vi "Imaging.vi"() -> ()   [LabVIEW 2015]
uses:
  <userlib>/atmcd64d.llb/Error Code Enum typedef.ctl
  <userlib>/atmcd64d.llb/AcquisitionMode_mode typedef.ctl
  <userlib>/atmcd64d.llb/HSSpeed_type typedef.ctl
  <userlib>/atmcd64d.llb/ReadMode_mode typedef.ctl
  <userlib>/atmcd64d.llb/TriggerMode_mode typedef.ctl
  <userlib>/atmcd64d.llb/Shutter_type typedef.ctl
  <userlib>/atmcd64d.llb/Shutter_mode typedef.ctl
  LiveImage.vi
panel:
  out "Intensity Graph":i32[][](graph)
  in  "Live Acquisition Start":bool
  in  "Set HS Speed":u16(ring) items=["17", "10", "5", "1"]
  out "#VS Speeds":i32
  in  "Acquisition Mode":T1=enum."Single Scan"
  in  "stop":bool
  out "status":T2
  out "minTemp":i32
  out "maxTemp":i32
  out "ypixels":i32
  out "xpixels":i32
  out "temperature":sgl
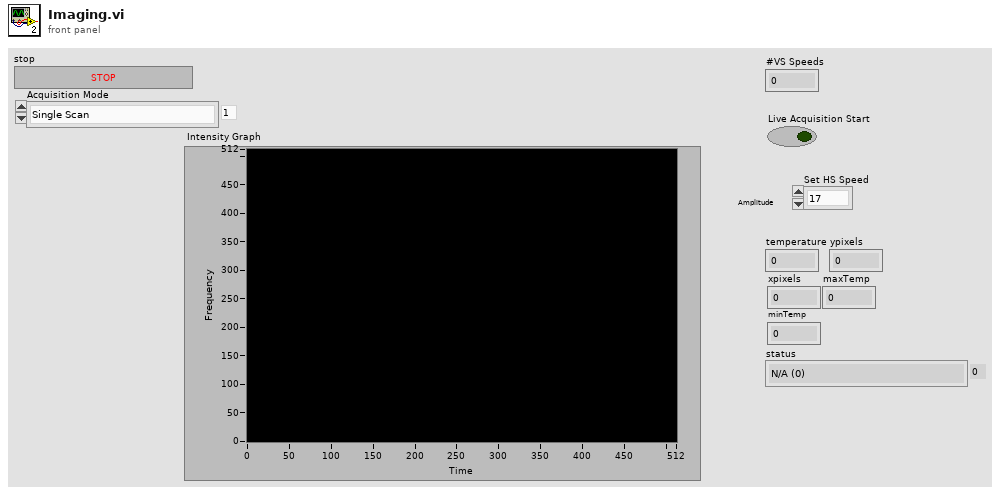
[diagram p1: front panel]
types:
  T1 = typedef "AcquisitionMode_mode typedef.ctl" = enum16{"Reserved (0)", "Single Scan", "Accumulate", "Kinetics", "Fast Kinetics", "Run Till Abort", "Reserved (6)", "Reserved (7)", "Reserved (8)", "Time Delayed Integration"}
  T2 = typedef "Error Code Enum typedef.ctl" = enum32{"N/A (0)", "DRV_ERROR_CODES", "DRV_SUCCESS", "DRV_VXDNOTINSTALLED", "DRV_ERROR_SCAN", "DRV_ERROR_CHECK_SUM", "DRV_ERROR_FILELOAD", "DRV_UNKNOWN_FUNC", "DRV_ERROR_VXD_INIT", "DRV_ERROR_ADDRESS", "DRV_ERROR_PAGELOCK", "DRV_ERROR_PAGEUNLOCK", "DRV_ERROR_BOARDTEST", "DRV_ERROR_ACK", "DRV_ERROR_UP_FIFO", "DRV_ERROR_PATTERN", "N/A (16)", "DRV_ACQUISITION_ERRORS", "DRV_ACQ_BUFFER", "DRV_ACQ_DOWNFIFO_FULL", "DRV_PROC_UNKONWN_INSTRUCTION", "DRV_ILLEGAL_OP_CODE", "DRV_KINETIC_TIME_NOT_MET", "DRV_ACCUM_TIME_NOT_MET", "DRV_NO_NEW_DATA", "N/A (25)", "DRV_SPOOLERROR", "N/A (27)", "N/A (28)", "N/A (29)", "N/A (30)", "N/A (31)", "N/A (32)", "DRV_TEMPERATURE_CODES", "DRV_TEMPERATURE_OFF", "DRV_TEMPERATURE_NOT_STABILIZED", "DRV_TEMPERATURE_STABILIZED", "DRV_TEMPERATURE_NOT_REACHED", "DRV_TEMPERATURE_OUT_RANGE", "DRV_TEMPERATURE_NOT_SUPPORTED", "DRV_TEMPERATURE_DRIFT", "N/A (41)", "N/A (42)", "N/A (43)", "N/A (44)", "N/A (45)", "N/A (46)", "N/A (47)", "N/A (48)", "DRV_GENERAL_ERRORS", "DRV_INVALID_AUX", "DRV_COF_NOTLOADED", "DRV_FPGAPROG", "DRV_FLEXERROR", "DRV_GPIBERROR", "N/A (55)", "N/A (56)", "N/A (57)", "N/A (58)", "N/A (59)", "N/A (60)", "N/A (61)", "N/A (62)", "N/A (63)", "DRV_DATATYPE", "DRV_DRIVER_ERRORS", "DRV_P1INVALID", "DRV_P2INVALID", "DRV_P3INVALID", "DRV_P4INVALID", "DRV_INIERROR", "DRV_COFERROR", "DRV_ACQUIRING", "DRV_IDLE", "DRV_TEMPCYCLE", "DRV_NOT_INITIALIZED", "DRV_P5INVALID", "DRV_P6INVALID", "DRV_INVALID_MODE", "DRV_INVALID_FILTER", "DRV_I2CERRORS", "DRV_I2CDEVNOTFOUND", "DRV_I2CTIMEOUT", "DRV_P7INVALID", "N/A (84)", "N/A (85)", "N/A (86)", "N/A (87)", "N/A (88)", "N/A (89)", "DRV_IOCERROR", "DRV_VRMVERSIONERROR"}
  T3 = typedef "Shutter_mode typedef.ctl" = enum16{"Auto", "Open", "Close", "N/A (3)", "Open FVB Series", "Open Any Series"}
  T4 = typedef "Shutter_type typedef.ctl" = enum16{"TTL Low", "TTL High"}
  T5 = typedef "TriggerMode_mode typedef.ctl" = enum16{"Internal", "External", "N/A (2)", "N/A (3)", "N/A (4)", "N/A (5)", "External Start", "External Exposure (Bulb)", "N/A (8)", "External FVB EM", "Software", "N/A (11)", "External Charge Shifting"}
  T6 = typedef "ReadMode_mode typedef.ctl" = enum16{"Full Vertical Binning", "Multi-Track", "Random-Track", "Single-Track", "Image"}
  T7 = typedef "HSSpeed_type typedef.ctl" = enum16{"EM Amp", "Conventional Amp"}
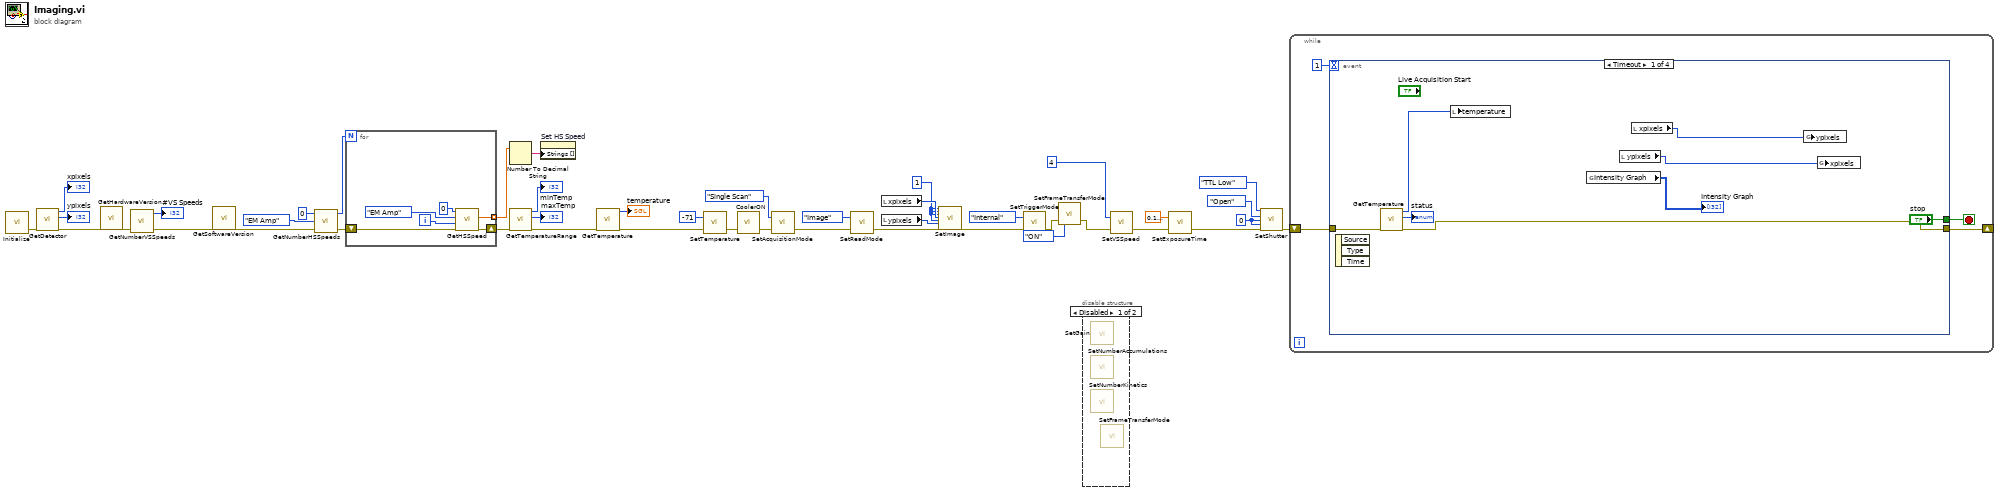
[diagram p0: block diagram]
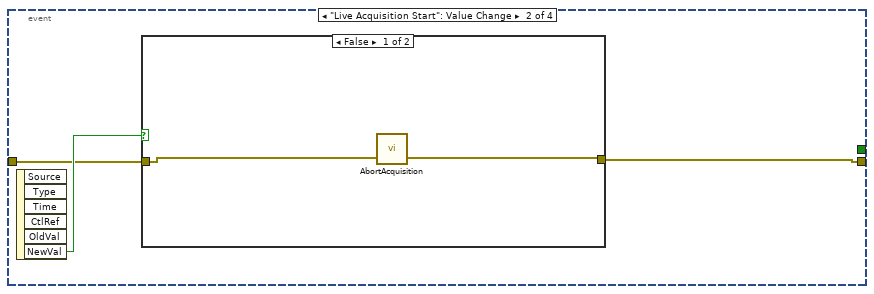
[diagram p3: hidden frame]
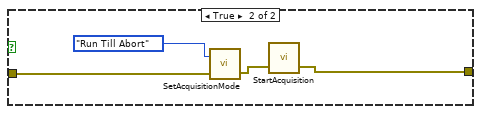
[diagram p4: hidden frame]
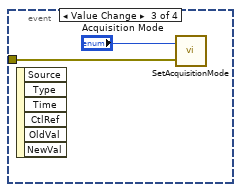
[diagram p5: hidden frame]
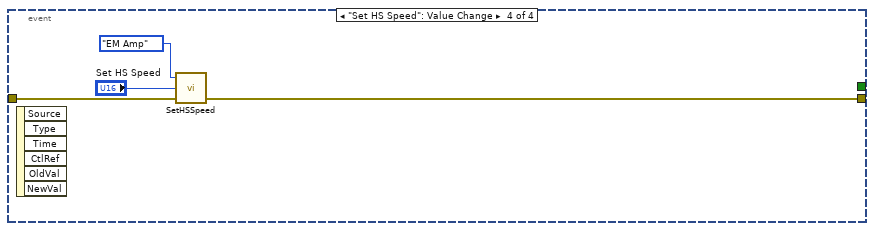
[diagram p6: hidden frame]
diagram:
  w5 = 0 ("closingtime")
  w11 = 1 ("hbin")
  n1 = call <userlib>:"Initialize.vi"() -> ("error out"=w42:errorcluster)  [unwired: 2 in, 1 out]
  n2 = call <userlib>:"GetDetector.vi"("error in (no error)"=w42) -> ("error out"=w41:errorcluster, "ypixels"=→"ypixels":i32, "xpixels"=→"xpixels":i32)  [unwired: 3 in, 1 out]
  n3 = call <userlib>:"GetHardwareVersion.vi"("error in (no error)"=w41) -> ("error out"=w38:errorcluster)  [unwired: 19 in, 7 out]
  n4 = call <userlib>:"GetNumberVSSpeeds.vi"("error in (no error)"=w38) -> ("error out"=w37:errorcluster, "number"=→"#VS Speeds":i32)  [unwired: 2 in, 1 out]
  n5 = call <userlib>:"GetSoftwareVersion.vi"("error in (no error)"=w37) -> ("error out"=w31:errorcluster)  [unwired: 19 in, 7 out]
  n6 = call <userlib>:"GetNumberHSSpeeds.vi"("error in (no error)"=w31, "type"=HSSpeed_type_typedef."EM Amp", "channel"=0) -> ("error out"=w30:errorcluster, "number"=w29:i32)  [unwired: 1 out]
  n7 = for {
    N: w29 -> [_]
    tunnel: [w48] -> w21 mode=indexing
    shift-right: [w46] -> w28
    shift-left: w30 -> [w49]
    i -> [w47]
    n8 = call <userlib>:"GetHSSpeed.vi"("error in (no error)"=w49, "index"=w47, "type"=HSSpeed_type_typedef."EM Amp", "channel"=0) -> ("error out"=w46:errorcluster, "speed"=w48:sgl)  [unwired: 1 in, 1 out]
  }
  n9 = Number To Decimal String(number=w21) -> (decimal integer string=w20:string[])  [unwired: 1 in]
  n10 = call <userlib>:"GetTemperatureRange.vi"("error in (no error)"=w28) -> ("error out"=w34:errorcluster, "maxTemp"=→"maxTemp":i32, "minTemp"=→"minTemp":i32)  [unwired: 3 in, 1 out]
  n11 = property on="Set HS Speed" class="Ring (strict)"("Strings []"=w20) -> ()  [unwired: 2 in, 2 out]
  n12 = call <userlib>:"GetTemperature.vi"("error in (no error)"=w34) -> ("error out"=w27:errorcluster, "temperature"=→"temperature":i32)  [unwired: 3 in, 2 out]
  n13 = call <userlib>:"SetTemperature.vi"("error in (no error)"=w27, "temperature"=-71) -> ("error out"=w26:errorcluster)  [unwired: 1 out]
  n14 = call <userlib>:"CoolerON.vi"("error in (no error)"=w26) -> ("error out"=w24:errorcluster)  [unwired: 1 in, 1 out]
  n15 = call <userlib>:"SetAcquisitionMode.vi"("error in (no error)"=w24, "mode"=AcquisitionMode_mode_typedef."Single Scan") -> ("error out"=w18:errorcluster)  [unwired: 1 out]
  n16 = call <userlib>:"SetReadMode.vi"("error in (no error)"=w18, "mode"=ReadMode_mode_typedef."Image") -> ("error out"=w14:errorcluster)  [unwired: 1 out]
  n17 = local read "xpixels"() -> (w12:i32)
  n18 = local read "ypixels"() -> (w10:i32)
  n19 = call <userlib>:"SetImage.vi"("hbin"=w11, "vbin"=w11, "hstart"=w11, "hend"=w12, "vstart"=w11, "vend"=w10, "error in (no error)"=w14) -> ("error out"=w13:errorcluster)  [unwired: 19 in, 1 out]
  n20 = call <userlib>:"SetTriggerMode.vi"("error in (no error)"=w13, "mode"=TriggerMode_mode_typedef."Internal") -> ("error out"=w3:errorcluster)  [unwired: 1 out]
  n21 = call <userlib>:"SetFrameTransferMode.vi"("error in (no error)"=w3, "mode"=enum16{"OFF", "ON"}."ON") -> ("error out"=w1:errorcluster)  [unwired: 1 out]
  n22 = disable-structure shown="Disabled" {
    frame Disabled {
      n23 = call <userlib>:"SetGain.vi"() -> ()  [unwired: 2 in, 2 out]
      n24 = call <userlib>:"SetNumberAccumulations.vi"() -> ()  [unwired: 2 in, 2 out]
      n25 = call <userlib>:"SetNumberKinetics.vi"() -> ()  [unwired: 2 in, 2 out]
      n26 = call <userlib>:"SetFrameTransferMode.vi"() -> ()  [unwired: 2 in, 2 out]
    }
    frame Enabled {
    }
  }
  n27 = call <userlib>:"SetVSSpeed.vi"("error in (no error)"=w1, "index"=4) -> ("error out"=w15:errorcluster)  [unwired: 1 out]
  n28 = call <userlib>:"SetExposureTime.vi"("error in (no error)"=w15, "time"=sgl 0.1) -> ("error out"=w9:errorcluster)  [unwired: 1 out]
  n29 = call <userlib>:"SetShutter.vi"("type"=Shutter_type_typedef."TTL Low", "mode"=Shutter_mode_typedef."Open", "closingtime"=w5, "openingtime"=w5, "error in (no error)"=w9) -> ("error out"=w8:errorcluster)  [unwired: 9 in, 1 out]
  n30 = while {
    shift-right: [w52] -> _
    shift-left: w8 -> [w53]
    stop <- w51 stop-if-true
    n31 = event shown="[0] Timeout" {
      selector: _ -> [_ _ _ _]
      dyn-events: _ -> [_ _ _ _]
      timeout: 1 -> [_ _ _ _]
      tunnel: w53 -> [w60 w63 w71 w75]
      tunnel: [w56 w62 _ w74] -> w52
      tunnel: ["stop" _ _ _] -> w51
      event Timeout {
        n32 = event-data() -> ()  [unwired: 1 in, 3 out]
        n33 = call <userlib>:"GetTemperature.vi"("error in (no error)"=w60) -> ("error out"=w56:errorcluster, "status"=→"status":T2, "temperature"=w58:i32)  [unwired: 3 in, 1 out]
        n34 = local write "temperature"(w58) -> ()
        n35 = global read "LiveImage.vi" "Intensity Graph"() -> (→"Intensity Graph":i32[][])
        n36 = local read "ypixels"() -> (w54:i32)
        n37 = local read "xpixels"() -> (w55:i32)
        n38 = global write "LiveImage.vi" "ypixels"(w55) -> ()
        n39 = global write "LiveImage.vi" "xpixels"(w54) -> ()
      }
      event "Live Acquisition Start": Value Change {
        n40 = event-data() -> ("NewVal"=w64:bool)  [unwired: 1 in, 5 out]
        n41 = case shown="False" w64 {
          tunnel: w63 -> [w66 w68]
          tunnel: [w65 w67] -> w62
          frame False {
            n42 = call <userlib>:"AbortAcquisition.vi"("error in (no error)"=w66) -> ("error out"=w65:errorcluster)  [unwired: 1 in, 1 out]
          }
          frame True {
            n43 = call <userlib>:"SetAcquisitionMode.vi"("error in (no error)"=w68, "mode"=AcquisitionMode_mode_typedef."Run Till Abort") -> ("error out"=w70:errorcluster)  [unwired: 1 out]
            n44 = call <userlib>:"StartAcquisition.vi"("error in (no error)"=w70) -> ("error out"=w67:errorcluster)  [unwired: 1 in, 1 out]
          }
        }
      }
      event Value Change {
        n45 = event-data() -> ()  [unwired: 1 in, 6 out]
        n46 = call <userlib>:"SetAcquisitionMode.vi"("error in (no error)"=w71, "mode"="Acquisition Mode") -> ()  [unwired: 2 out]
      }
      event "Set HS Speed": Value Change {
        n47 = event-data() -> ()  [unwired: 1 in, 6 out]
        n48 = call <userlib>:"SetHSSpeed.vi"("error in (no error)"=w75, "index"="Set HS Speed", "type"=HSSpeed_type_typedef."EM Amp") -> ("error out"=w74:errorcluster)  [unwired: 1 in, 1 out]
      }
    }
  }
